vi "Next Song.vi"(0 "reference in":refnum<class "MusicPlayer.lvclass">, 11 "Error In":errorcluster) -> (4 "reference out":refnum<class "MusicPlayer.lvclass">, 15 "Error Out":errorcluster)   [LabVIEW 2022 SP3, in "MusicPlayer.lvclass"]
uses:
  MusicPlayer.lvclass
  MusicPlayer.lvclass/MusicPlayer.ctl
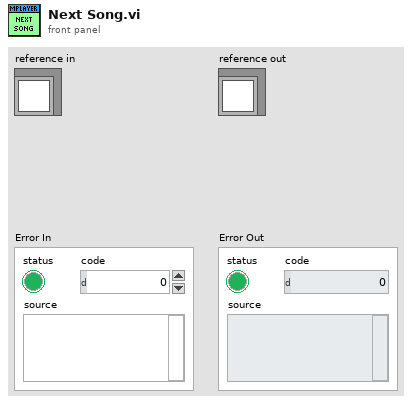
[diagram p1: front panel]
types:
  T1 = typedef "MusicPlayer.lvclass/ObjectAttributes.ctl" = cluster{"MediaPlayer":refnum<k7>, "Playlist":path[], "Index":u32}
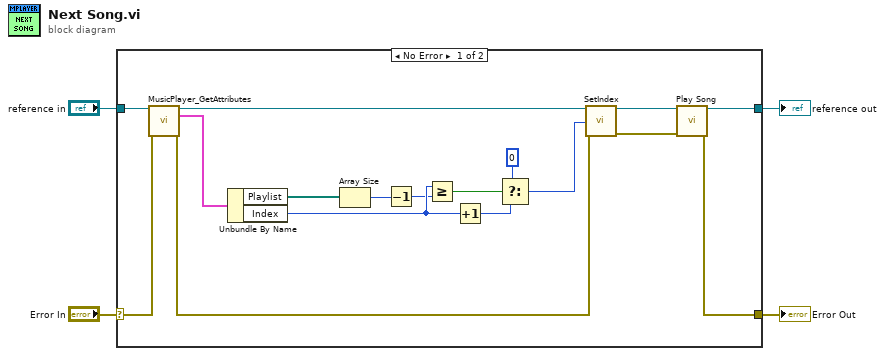
[diagram p0: block diagram]
diagram:
  n1 = case shown="No Error" "Error In" {
    selector: "Error In" -> [w21 w23]
    tunnel: [w5 w23] -> w3
    tunnel: [w9 w22] -> w1
    tunnel: "reference in" -> [w19 w22]
    frame No Error {
      n2 = call "MusicPlayer_GetAttributes.vi"("reference in"=w19, "error in (no error)"=w21) -> ("reference out"=w18:refnum<class "MusicPlayer.lvclass">, "Data"=w20:T1, "error out"=w7:errorcluster)  [unwired: 10 in, 1 out]
      n3 = Unbundle By Name(w20) -> ("Playlist"=w17:path[], "Index"=w14:u32)
      n4 = Array Size(array=w17) -> (size(s)=w16:i32)
      n5 = Decrement(x=w16) -> (x-1=w12:i32)
      n6 = Greater Or Equal?(x=w14, y=w12) -> (x >= y?=w15:bool)
      n7 = Increment(x=w14) -> (x+1=w13:u32)
      n8 = Select(t=u32 0, s=w15, f=w13) -> (s? t:f=w8:u32)
      n9 = call "SetIndex.vi"("reference in"=w18, "Index"=w8, "Error In"=w7) -> ("reference out"=w10:refnum<class "MusicPlayer.lvclass">, "Error Out"=w6:errorcluster)  [unwired: 11 in]
      n10 = call-dynamic "Play Song.vi"("reference in"=w10, "Error In"=w6) -> ("reference out"=w9:refnum<class "MusicPlayer.lvclass">, "Error Out"=w5:errorcluster)  [unwired: 12 in]
    }
    frame Error {
    }
  }
  "Error Out" <- w3
  "reference out" <- w1
